vi "Variable list Driller digital.vi"() -> (6 "Variant":variant, 10 "Array":T1[](array[typedef]))   [LabVIEW 2011]
uses:
  Measurments Handling/Fixed Digital Channel Definition.ctl
  Measurments Handling/Update frequensies.ctl
  Measurments Handling/Channel catagory Enum.ctl
  Variable List Driller Digital.ctl
  Extende dchannel identefier for driller Digtal.ctl
  <vilib>/Utility/VariantDataType/GetNumericInfo.vi
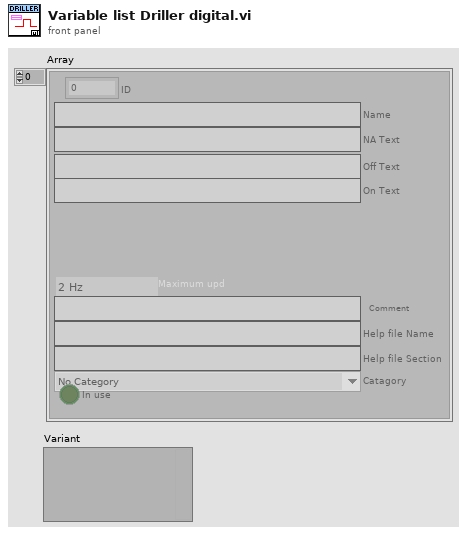
[diagram p1: front panel]
types:
  T1 = typedef "Fixed Digital Channel Definition.ctl" = cluster{"ID":u16, "Name":string, "NA Text":string, "Off Text":string, "On Text":string, "Maximum upd":T2, "Comment":string, "Help file Name":string, "Help file Section ":string, "Catagory":T3, "In use":bool}
  T2 = typedef "Update frequensies.ctl" = enum16{"2 Hz", "1 Hz", "0.1 Hz"}
  T3 = typedef "Channel catagory Enum.ctl" = enum16{"No Category", "Power", "Temperature", "Pressure"}
  T4 = typedef "Extende dchannel identefier for driller Digtal.ctl" = cluster{"Name":T5, "Variable Defenition":T1}
  T5 = typedef "Variable List Driller Digital.ctl" = enum16{"Tool Relay 1", "Tool Relay 2", "Tool node pressure 1", "Tool node pressure 2", "Tool node solenoid", "Tool node motor", "Tool High G Monitoring", "Tool High G Recording", "Tool High G Data ready", "Tool error Controller", "Tool error Pressure 1", "Tool error Pressure 2", "Tool error Solenoid", "Tool stopped Controller", "Tool stopped Pressure 1", "Tool stopped Pressure 2", "Tool stopped Solenoid", "Stroke Moving Out", "Stroke Moving Inn", "Oil filling mode", "Mill Bit Direction", "Reserved", "Tool Solenoid 1", "Tool Solenoid 2", "Tool Solenoid 3", "Position control", "Anchor"}
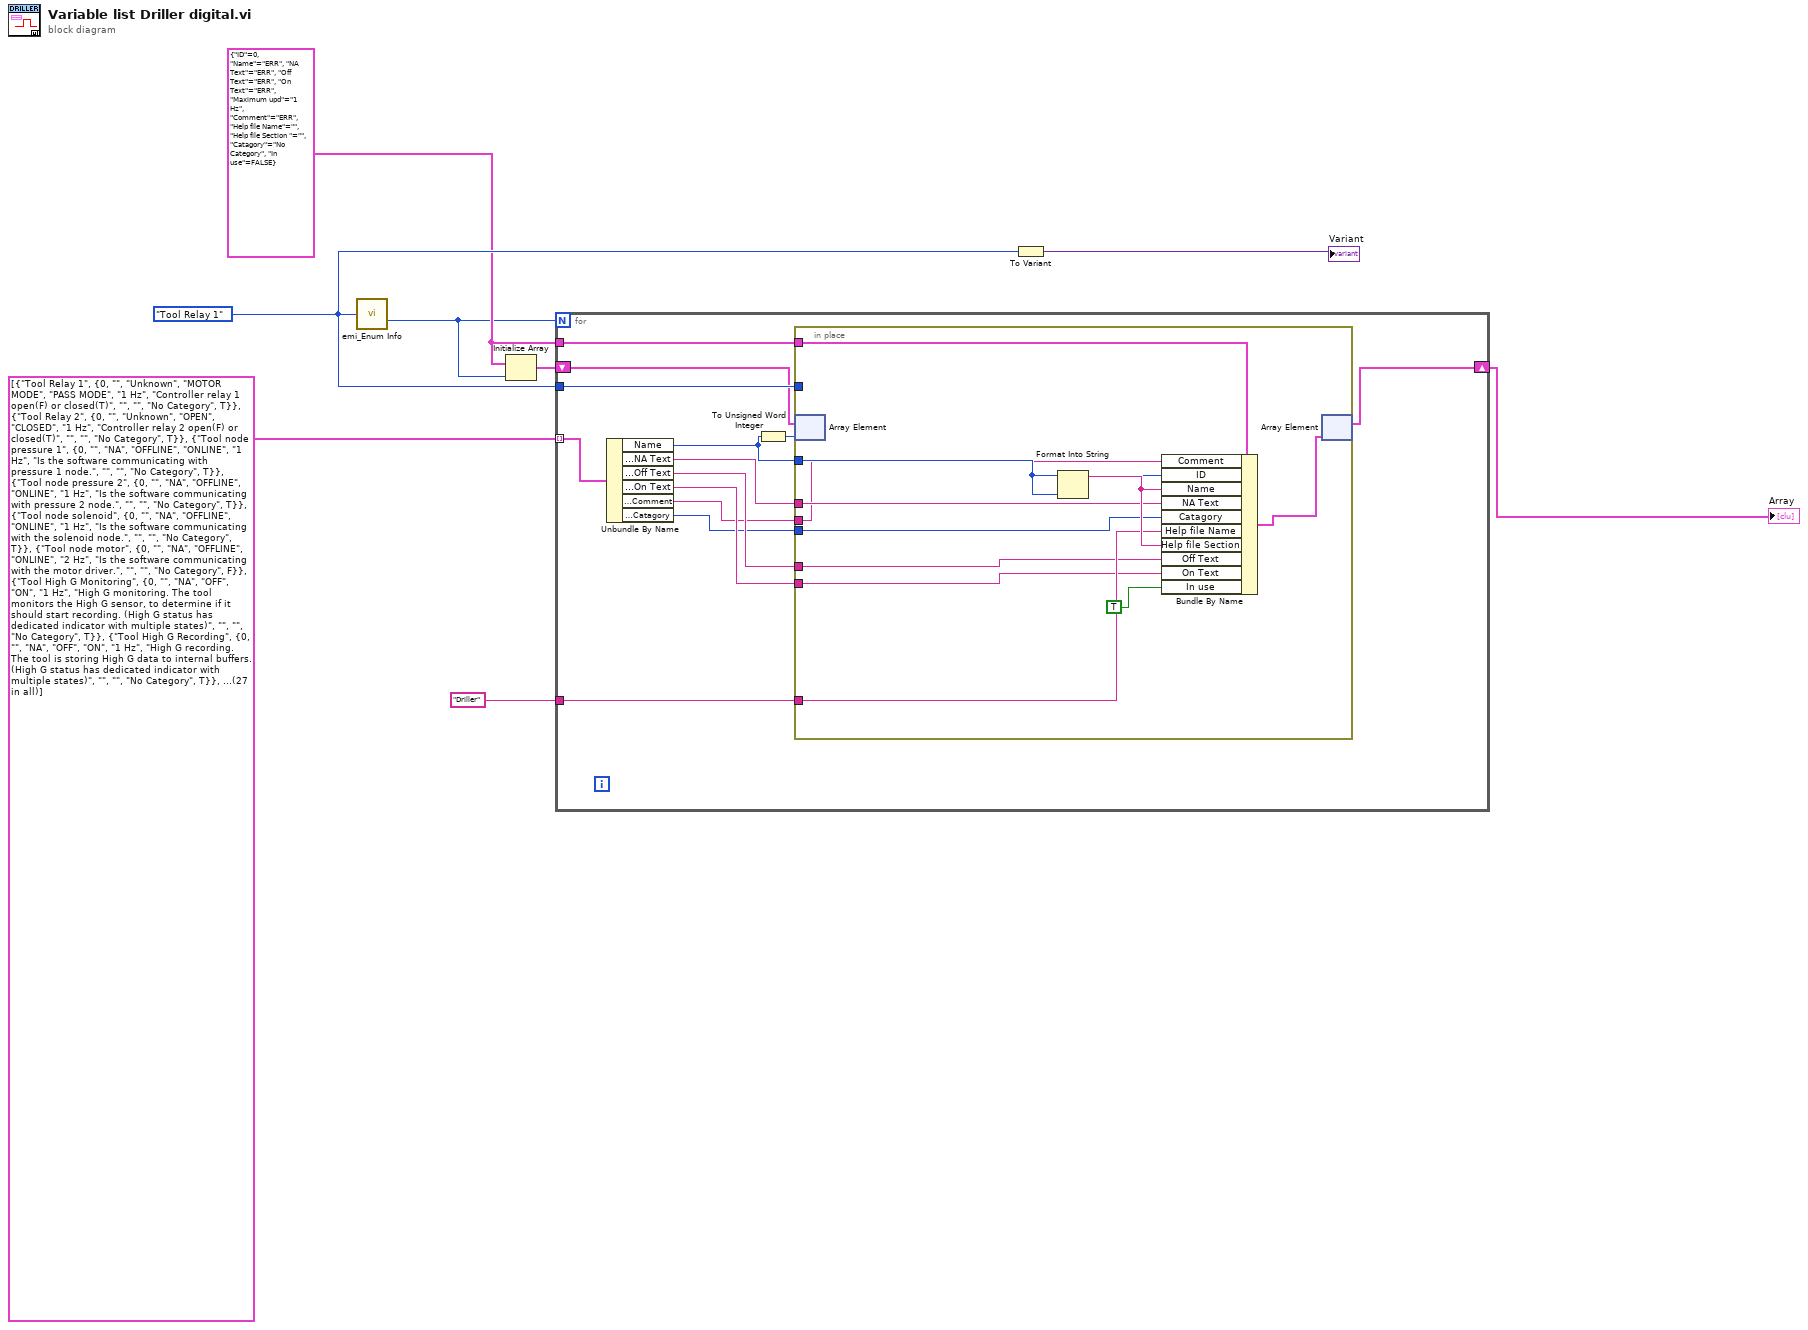
[diagram p0: block diagram]
diagram:
  w4 = T1 {"ID"=0, "Name"="ERR", "NA Text"="ERR", "Off Text"="ERR", "On Text"="ERR", "Maximum upd"=enum."1 Hz", "Comment"="ERR", "Help file Name"="", "Help file Section "="", "Catagory"=enum."No Category", "In use"=FALSE} ("Variable Defenition")
  w7 = Variable_List_Driller_Digital."Tool Relay 1" ("Action")
  n1 = call "emi_Enum Info.vi"("Enum"=w7) -> ("Numb Elements"=w3:i32)  [unwired: 11 in, 3 out]
  n2 = Initialize Array(w4, w3) -> (w2:T1[])
  n3 = for {
    N: w3 -> [_]
    tunnel: w7 -> [w21]
    tunnel: w4 -> [w10]
    tunnel: "Driller" -> [w20]
    tunnel: T4[] [{"Name"=enum."Tool Relay 1", "Variable Defenition"={"ID"=0, "Name"="", "NA Text"="Unknown", "Off Text"="MOTOR MODE", "On Text"="PASS MODE", "Maximum upd"=enum."1 Hz", "Comment"="Controller relay 1 open(F) or closed(T)", "Help file Name"="", "Help file Section "="", "Catagory"=enum."No Category", "In use"=TRUE}}, {"Name"=enum."Tool Relay 2", "Variable Defenition"={"ID"=0, "Name"="", "NA Text"="Unknown", "Off Text"="OPEN", "On Text"="CLOSED", "Maximum upd"=enum."1 Hz", "Comment"="Controller relay 2 open(F) or closed(T)", "Help file Name"="", "Help file Section "="", "Catagory"=enum."No Category", "In use"=TRUE}}, {"Name"=enum."Tool node pressure 1", "Variable Defenition"={"ID"=0, "Name"="", "NA Text"="NA", "Off Text"="OFFLINE", "On Text"="ONLINE", "Maximum upd"=enum."1 Hz", "Comment"="Is the software communicating with pressure 1 node.", "Help file Name"="", "Help file Section "="", "Catagory"=enum."No Category", "In use"=TRUE}}, {"Name"=enum."Tool node pressure 2", "Variable Defenition"={"ID"=0, "Name"="", "NA Text"="NA", "Off Text"="OFFLINE", "On Text"="ONLINE", "Maximum upd"=enum."1 Hz", "Comment"="Is the software communicating with pressure 2 node.", "Help file Name"="", "Help file Section "="", "Catagory"=enum."No Category", "In use"=TRUE}}, {"Name"=enum."Tool node solenoid", "Variable Defenition"={"ID"=0, "Name"="", "NA Text"="NA", "Off Text"="OFFLINE", "On Text"="ONLINE", "Maximum upd"=enum."1 Hz", "Comment"="Is the software communicating with the solenoid node.", "Help file Name"="", "Help file Section "="", "Catagory"=enum."No Category", "In use"=TRUE}}, {"Name"=enum."Tool node motor", "Variable Defenition"={"ID"=0, "Name"="", "NA Text"="NA", "Off Text"="OFFLINE", "On Text"="ONLINE", "Maximum upd"=enum."2 Hz", "Comment"="Is the software communicating with the motor driver.", "Help file Name"="", "Help file Section "="", "Catagory"=enum."No Category", "In use"=FALSE}}, {"Name"=enum."Tool High G Monitoring", "Variable Defenition"={"ID"=0, "Name"="", "NA Text"="NA", "Off Text"="OFF", "On Text"="ON", "Maximum upd"=enum."1 Hz", "Comment"="High G monitoring. The tool monitors the High G sensor, to determine if it should start recording. (High G status has dedicated indicator with multiple states)", "Help file Name"="", "Help file Section "="", "Catagory"=enum."No Category", "In use"=TRUE}}, {"Name"=enum."Tool High G Recording", "Variable Defenition"={"ID"=0, "Name"="", "NA Text"="NA", "Off Text"="OFF", "On Text"="ON", "Maximum upd"=enum."1 Hz", "Comment"="High G recording. The tool is storing High G data to internal buffers. (High G status has dedicated indicator with multiple states)", "Help file Name"="", "Help file Section "="", "Catagory"=enum."No Category", "In use"=TRUE}}, {"Name"=enum."Tool High G Data ready", "Variable Defenition"={"ID"=0, "Name"="", "NA Text"="NA", "Off Text"="NO DATA", "On Text"="DATA READY", "Maximum upd"=enum."1 Hz", "Comment"="There is High G data stored in the tools internal buffers. (High G status has dedicated indicator with multiple states)", "Help file Name"="", "Help file Section "="", "Catagory"=enum."No Category", "In use"=TRUE}}, {"Name"=enum."Tool error Controller", "Variable Defenition"={"ID"=0, "Name"="", "NA Text"="Unknown", "Off Text"="OK", "On Text"="ERROR", "Maximum upd"=enum."1 Hz", "Comment"="Controller node has an error.\nTo clear an error, or gather more details when an error occurs, see \"Detail view\" in main menu.", "Help file Name"="", "Help file Section "="", "Catagory"=enum."No Category", "In use"=TRUE}}, {"Name"=enum."Tool error Pressure 1", "Variable Defenition"={"ID"=0, "Name"="", "NA Text"="Unknown", "Off Text"="OK", "On Text"="ERROR", "Maximum upd"=enum."1 Hz", "Comment"="Pressure node 1 has an error.\nTo clear an error, or gather more details when an error occurs, see \"Detail view\" in main menu.", "Help file Name"="", "Help file Section "="", "Catagory"=enum."No Category", "In use"=TRUE}}, {"Name"=enum."Tool error Pressure 2", "Variable Defenition"={"ID"=0, "Name"="", "NA Text"="Unknown", "Off Text"="OK", "On Text"="ERROR", "Maximum upd"=enum."1 Hz", "Comment"="Pressure node 2 has an error.\nTo clear an error, or gather more details when an error occurs, see \"Detail view\" in main menu.", "Help file Name"="", "Help file Section "="", "Catagory"=enum."No Category", "In use"=TRUE}}, {"Name"=enum."Tool error Solenoid", "Variable Defenition"={"ID"=0, "Name"="", "NA Text"="Unknown", "Off Text"="OK", "On Text"="ERROR", "Maximum upd"=enum."1 Hz", "Comment"="Solenoid node  has an error.\nTo clear an error, or gather more details when an error occurs, see \"Detail view\" in main menu.", "Help file Name"="", "Help file Section "="", "Catagory"=enum."No Category", "In use"=TRUE}}, {"Name"=enum."Tool stopped Controller", "Variable Defenition"={"ID"=0, "Name"="", "NA Text"="Unknown", "Off Text"="RUNNING", "On Text"="STOPPED", "Maximum upd"=enum."1 Hz", "Comment"="Controller node has been stopped by stop command, or connection timeout.", "Help file Name"="", "Help file Section "="", "Catagory"=enum."No Category", "In use"=TRUE}}, {"Name"=enum."Tool stopped Pressure 1", "Variable Defenition"={"ID"=0, "Name"="", "NA Text"="Unknown", "Off Text"="RUNNING", "On Text"="STOPPED", "Maximum upd"=enum."1 Hz", "Comment"="Pressure node 1 has been stopped by stop command, or connection timeout.", "Help file Name"="", "Help file Section "="", "Catagory"=enum."No Category", "In use"=TRUE}}, {"Name"=enum."Tool stopped Pressure 2", "Variable Defenition"={"ID"=0, "Name"="", "NA Text"="Unknown", "Off Text"="RUNNING", "On Text"="STOPPED", "Maximum upd"=enum."1 Hz", "Comment"="Pressure node 2 has been stopped by stop command, or connection timeout.", "Help file Name"="", "Help file Section "="", "Catagory"=enum."No Category", "In use"=TRUE}}, {"Name"=enum."Tool stopped Solenoid", "Variable Defenition"={"ID"=0, "Name"="", "NA Text"="Unknown", "Off Text"="RUNNING", "On Text"="STOPPED", "Maximum upd"=enum."1 Hz", "Comment"="Solenoid node has been stopped by stop command, or connection timeout.", "Help file Name"="", "Help file Section "="", "Catagory"=enum."No Category", "In use"=TRUE}}, {"Name"=enum."Stroke Moving Out", "Variable Defenition"={"ID"=0, "Name"="", "NA Text"="NA", "Off Text"="STILL", "On Text"="MOVING", "Maximum upd"=enum."1 Hz", "Comment"="Stroke has been detected as moving out.", "Help file Name"="", "Help file Section "="", "Catagory"=enum."No Category", "In use"=TRUE}}, {"Name"=enum."Stroke Moving Inn", "Variable Defenition"={"ID"=0, "Name"="", "NA Text"="NA", "Off Text"="STILL", "On Text"="MOVING", "Maximum upd"=enum."1 Hz", "Comment"="troke has been detected as moving inn.", "Help file Name"="", "Help file Section "="", "Catagory"=enum."No Category", "In use"=TRUE}}, {"Name"=enum."Oil filling mode", "Variable Defenition"={"ID"=0, "Name"="", "NA Text"="NA", "Off Text"="OFF", "On Text"="OIL FILLING", "Maximum upd"=enum."1 Hz", "Comment"="Oil filling mode detected", "Help file Name"="", "Help file Section "="", "Catagory"=enum."No Category", "In use"=TRUE}}, {"Name"=enum."Mill Bit Direction", "Variable Defenition"={"ID"=0, "Name"="", "NA Text"="NA", "Off Text"="DIR A", "On Text"="DIR B", "Maximum upd"=enum."1 Hz", "Comment"="Mill Bit direction", "Help file Name"="", "Help file Section "="", "Catagory"=enum."No Category", "In use"=TRUE}}, {"Name"=enum."Reserved", "Variable Defenition"={"ID"=0, "Name"="", "NA Text"="NA", "Off Text"="-", "On Text"="-", "Maximum upd"=enum."1 Hz", "Comment"="Reserved", "Help file Name"="", "Help file Section "="", "Catagory"=enum."No Category", "In use"=TRUE}}, {"Name"=enum."Tool Solenoid 1", "Variable Defenition"={"ID"=0, "Name"="", "NA Text"="UNKNOWN", "Off Text"="OPEN", "On Text"="CLOSED", "Maximum upd"=enum."1 Hz", "Comment"="Solenoid 1 state", "Help file Name"="", "Help file Section "="", "Catagory"=enum."No Category", "In use"=TRUE}}, {"Name"=enum."Tool Solenoid 2", "Variable Defenition"={"ID"=0, "Name"="", "NA Text"="UNKNOWN", "Off Text"="OPEN", "On Text"="CLOSED", "Maximum upd"=enum."2 Hz", "Comment"="Solenoid 2 state", "Help file Name"="", "Help file Section "="", "Catagory"=enum."No Category", "In use"=FALSE}}, {"Name"=enum."Tool Solenoid 3", "Variable Defenition"={"ID"=0, "Name"="", "NA Text"="UNKNOWN", "Off Text"="OPEN", "On Text"="CLOSED", "Maximum upd"=enum."2 Hz", "Comment"="Solenoid 3 state", "Help file Name"="", "Help file Section "="", "Catagory"=enum."No Category", "In use"=FALSE}}, {"Name"=enum."Position control", "Variable Defenition"={"ID"=0, "Name"="", "NA Text"="NA", "Off Text"="-", "On Text"="POS CONT", "Maximum upd"=enum."2 Hz", "Comment"="", "Help file Name"="", "Help file Section "="", "Catagory"=enum."No Category", "In use"=FALSE}}, {"Name"=enum."Anchor", "Variable Defenition"={"ID"=0, "Name"="", "NA Text"="NA", "Off Text"="OFF", "On Text"="ACTIVE", "Maximum upd"=enum."2 Hz", "Comment"="", "Help file Name"="", "Help file Section "="", "Catagory"=enum."No Category", "In use"=FALSE}}] ("Array 2") -> [w19] mode=indexing
    shift-right: [w16] -> w1
    shift-left: w2 -> [w18]
    n4 = Unbundle By Name(w19) -> ("Name"=w12:T5, "Variable Defenition.NA Text"=w15:string, "Variable Defenition.Off Text"=w14:string, "Variable Defenition.On Text"=w13:string, "Variable Defenition.Comment"=w11:string, "Variable Defenition.Catagory"=w9:T3)
    n5 = To Unsigned Word Integer(number=w12) -> (unsigned 16bit integer=w17:u16)
    n6 = in-place {
      in-place-border: w21 -> [_]
      in-place-border: w12 -> [w26]
      in-place-border: w20 -> [w30]
      in-place-border: w15 -> [w29]
      in-place-border: w14 -> [w28]
      in-place-border: w13 -> [w27]
      in-place-border: w11 -> [w25]
      in-place-border: w10 -> [w23]
      in-place-border: w9 -> [w22]
      n7 = in-place-array #1(w18, w17) -> ()  [unwired: 1 out]
      n8 = Format Into String(w26) -> (resulting string=w32:string)  [unwired: 3 in, 1 out]
      n9 = Bundle By Name(cluster=w23, "Comment"=w25, "ID"=w26, "Name"=w32, "NA Text"=w29, "Catagory"=w22, "Help file Name"=w30, "Help file Section"=w32, "Off Text"=w28, "On Text"=w27, "In use"=TRUE) -> (w24:T1)
      n10 = in-place-array #1(w24) -> (w16:T1[])  [unwired: 1 out]
    }
  }
  "Array" <- w1
  n11 = To Variant(anything=w7) -> (Variant=→"Variant":variant)
